vi "Set Graphics.vi"(8 "error in (no error)":errorcluster, 10 "Graphics":refnum<class "Graphic.lvclass">[](array[class]), 11 "Canvas in":refnum<class "Canvas.lvclass">) -> (0 "error out":errorcluster, 3 "Canvas out":refnum<class "Canvas.lvclass">)   [LabVIEW 2015, in "Canvas.lvclass"]
uses:
  Canvas.lvclass
  Graphic/Graphic.lvclass
  Canvas.lvclass/Canvas.ctl
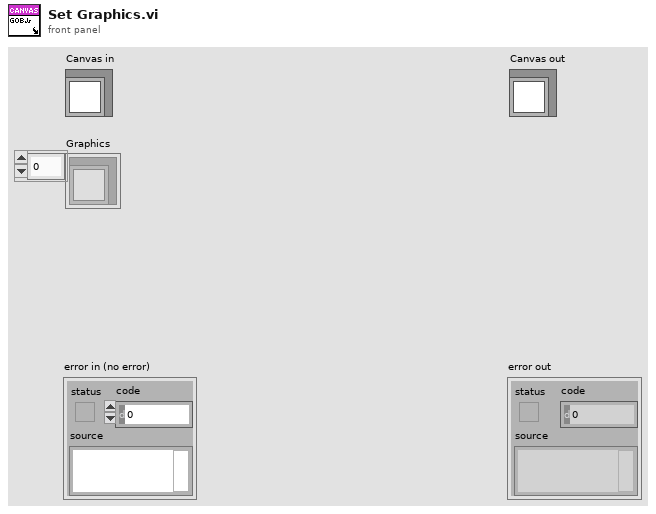
[diagram p1: front panel]
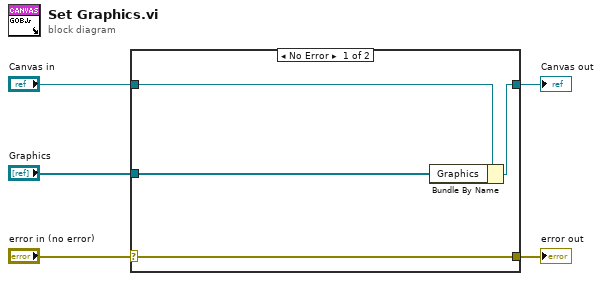
[diagram p0: block diagram]
diagram:
  n1 = case shown="No Error" "error in (no error)" {
    selector: "error in (no error)" -> [w9 w10]
    tunnel: [w9 w10] -> w4
    tunnel: [w7 w11] -> w2
    tunnel: "Canvas in" -> [w8 w11]
    tunnel: "Graphics" -> [w6 _]
    frame No Error {
      n2 = Bundle By Name(cluster=w8, "Graphics"=w6) -> (w7:refnum<class "Canvas.lvclass">)
    }
    frame Error {
    }
  }
  "error out" <- w4
  "Canvas out" <- w2
